vi "Save TS DAC Configuration.vi"(8 "error in":errorcluster, 11 "Generic Test Stand in":refnum<class "Generic Test Stand.lvclass">) -> (0 "error out":errorcluster, 3 "Generic Test Stand out":refnum<class "Generic Test Stand.lvclass">)   [LabVIEW 2019, in "Generic Test Stand.lvclass"]
uses:
  Generic Test Stand.lvclass
  Generic Test Stand.lvclass/Generic Test Stand.ctl
  DAC/DAC.lvclass
  <vilib>/Utility/config.llb/NI_LVConfig.lvlib
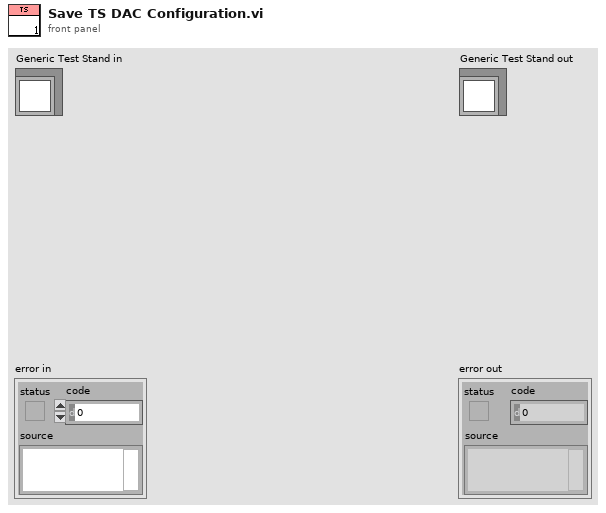
[diagram p1: front panel]
types:
  T1 = typedef "NI_LVConfig.lvlib/Config Data RefNum.ctl" = refnum<k1>
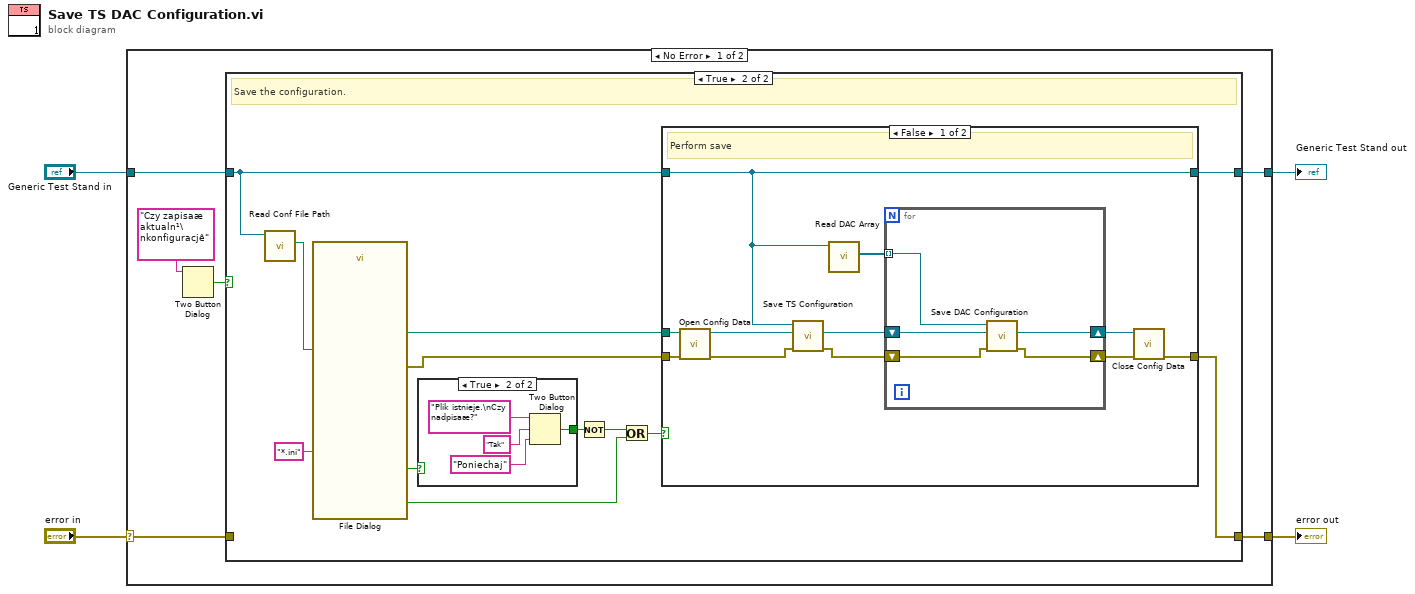
[diagram p0: block diagram]
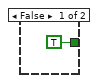
[diagram p3: hidden frame]
diagram:
  n1 = case shown="No Error" "error in" {
    selector: "error in" -> [w5 w49]
    tunnel: [w6 w49] -> w3
    tunnel: [w7 w48] -> w1
    tunnel: "Generic Test Stand in" -> [w8 w48]
    frame No Error {
      n2 = Two Button Dialog(message="Czy zapisaæ aktualn¹\nkonfiguracjê") -> (T button?=w10:bool)  [unwired: 2 in]
      n3 = case shown="True" w10 {
        tunnel: w8 -> [w12 w15]
        tunnel: [w12 w16] -> w7
        tunnel: [w11 w13] -> w6
        tunnel: w5 -> [w11 _]
        frame False {
          # "Save aborted."
        }
        frame True {
          # "Save the configuration."
          n4 = call "Read Conf File Path.vi"("Generic Test Stand in"=w15) -> ("Conf File Path"=w14:path)  [unwired: 8 in, 2 out]
          n5 = call "File Dialog"("start path"=w14, "pattern (all files)"="*.ini") -> ("selected path"=w24:path, "exists"=w21:bool, "cancelled"=w17:bool, "error out"=w23:errorcluster)  [unwired: 10 in]
          n6 = case shown="True" w21 {
            tunnel: [TRUE ("T button?") w26] -> w20
            frame False {
            }
            frame True {
              n7 = Two Button Dialog(message="Plik istnieje.\nCzy nadpisaæ?", 1:"Poniechaj" ("F button name (\"Cancel\")"), 2:"Tak" ("T button name (\"OK\")")) -> (T button?=w26:bool)
            }
          }
          n8 = Not(x=w20) -> (.not. x?=w18:bool)
          n9 = Or(x=w18, y=w17) -> (x .or. y?=w19:bool)
          n10 = case shown="False" w19 {
            tunnel: [w40 w46] -> w13
            tunnel: w24 -> [w39 _]
            tunnel: w23 -> [w38 w46]
            tunnel: w15 -> [w32 w47]
            tunnel: [w32 w47] -> w16
            frame False {
              # "Perform save"
              n11 = call <vilib>:"Open Config Data.vi"("error in (no error)"=w38, "configuration file path"=w39) -> ("error out"=w34:errorcluster, "refnum"=w31:T1)  [unwired: 7 in, 1 out]
              n12 = call-dynamic "Save TS Configuration.vi"("error in"=w34, "Config File refnum in"=w31, "Generic Test Stand in"=w32) -> ("error out"=w33:errorcluster, "Config File refnum out"=w30:T1)  [unwired: 6 in, 1 out]
              n13 = call "Read DAC Array.vi"("Generic Test Stand in"=w32) -> ("DAC Array"=w37:refnum<class "DAC.lvclass">[])  [unwired: 8 in, 2 out]
              n14 = for {
                tunnel: w37 -> [w45] mode=indexing
                shift-right: [w43] -> w36
                shift-left: w30 -> [w44]
                shift-right: [w41] -> w35
                shift-left: w33 -> [w42]
                n15 = call-dynamic "Save DAC Configuration.vi"("error in"=w42, "Config File refnum in"=w44, "DAC in"=w45) -> ("error out"=w41:errorcluster, "Config File refnum out"=w43:T1)  [unwired: 6 in, 1 out]
              }
              n16 = call <vilib>:"Close Config Data.vi"("error in (no error)"=w35, "refnum"=w36) -> ("error out"=w40:errorcluster)  [unwired: 8 in, 1 out]
            }
            frame True {
              # "Save cancelled"
            }
          }
        }
      }
    }
    frame Error {
    }
  }
  "error out" <- w3
  "Generic Test Stand out" <- w1
